vi "Host Main.vi"() -> ()   [LabVIEW 2017]
doc: "This application launches and executes the Tag Bus Data framework configuration for the specified target alias. This is a simple example of the framework API functions, but may also be a suitable starting point for a Host UI or Thick Client that is running a local version of the framework."
uses:
  <vilib>/NI/Module Execution Interface/Engine Runtime/Execution States.ctl
  <vilib>/NI/Module Execution Interface/Engine Runtime/Fault.ctl
  <vilib>/NI/Tag Bus Module Framework/runtime/error classification.ctl
  <vilib>/NI/Current Value Table/DataTypes/Double_Read.vi
  <vilib>/NI/Current Value Table/Type to Enum.vi
  <vilib>/NI/Current Value Table/DataTypes/Double_Type To Enum.vi
  <vilib>/NI/Current Value Table/FGVs/CVT Globals.vi
  <vilib>/NI/Current Value Table/FGVs/Tag Memory.vi
  <vilib>/NI/Current Value Table/Memory Block.vi
  <vilib>/NI/Current Value Table/DataTypes/Double_Memory Block.vi
  <vilib>/NI/Module Execution Interface/Engine Runtime/Engine Runtime Interface.lvclass
  <vilib>/NI/DCAF/Tag Editor Core/Framework Configuration Classes/target runtime/PL_Target Runtime.lvclass
  <vilib>/NI/Tag Bus Module Framework/runtime/TBM module execution interface.lvclass
  <vilib>/NI/Current Value Table/Current Value Table.lvlib
panel:
  out "Value":dbl
  out "engine status":T4(array[cluster])
  in  "stop":bool
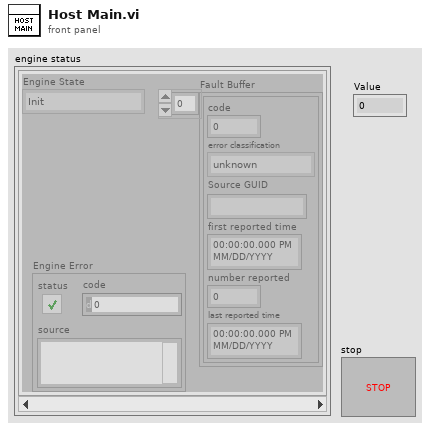
[diagram p1: front panel]
types:
  T1 = typedef "Engine Runtime Interface.lvclass/Execution States.ctl" = enum16{"Init", "Pre-Operational", "Safe-Operational", "Operational", "Stopped"}
  T2 = typedef "Engine Runtime Interface.lvclass/Fault.ctl" = cluster{"code":i32, "error classification":T3, "Source GUID":string, "first reported time":timestamp, "number reported":u32, "last reported time":timestamp}
  T3 = typedef "TBM module execution interface.lvclass/error classification.ctl" = enum16{"unknown", "none", "trivial", "recoverable", "critical"}
  T4 = cluster{"Engine State":T1, "Fault Buffer":T2[], "Engine Error":errorcluster}[]
  T5 = cluster{"Engine State":T1, "Fault Buffer":T2[], "Engine Error":errorcluster}
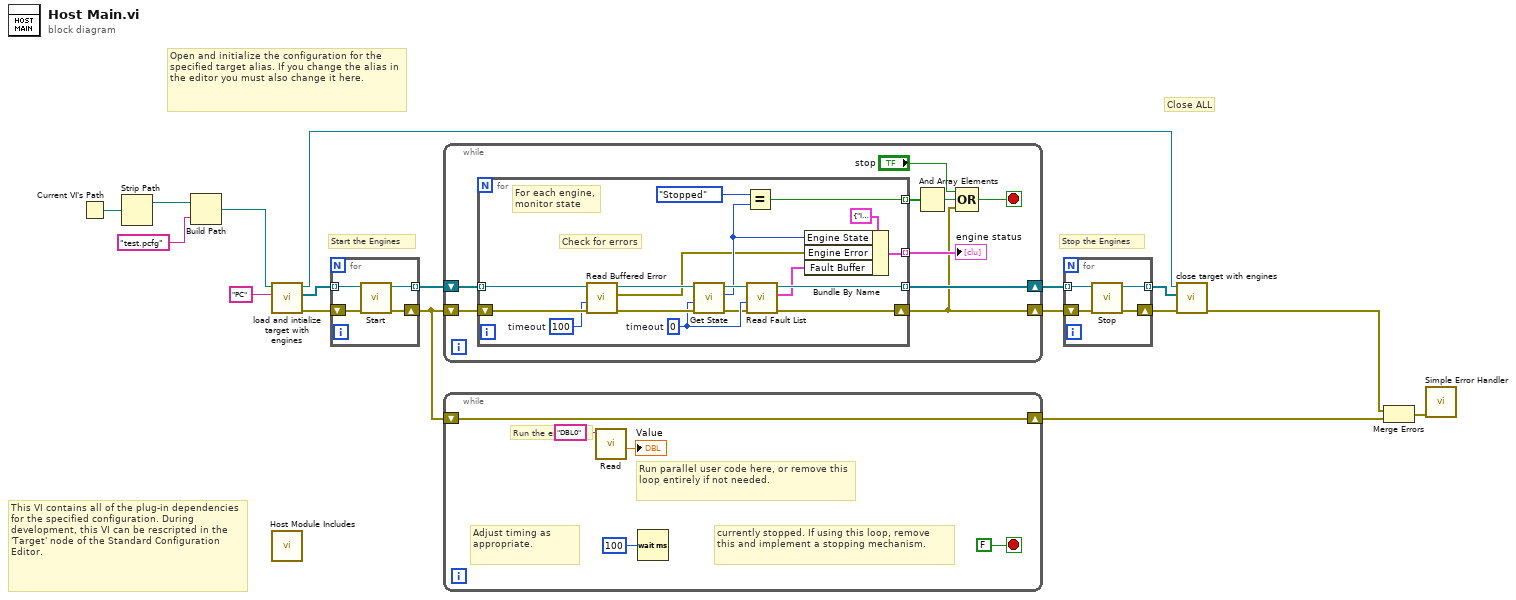
[diagram p0: block diagram]
diagram:
  # "Start the Engines"
  # "Open and initialize the configuration for the specified target alias. If you change the alias in the editor you must also change it here."
  # "Close ALL"
  # "Stop the Engines"
  # "This VI contains all of the plug-in dependencies for the specified configuration. During development, this VI can be rescripted in the 'Target' node of the Standard Configuration Editor."
  # "Run the engines"
  n1 = Current VI's Path() -> (path=w4:path)
  n2 = Strip Path(path=w4) -> (stripped path=w3:path)  [unwired: 1 out]
  n3 = Build Path(base path=w3, name or relative path="test.pcfg") -> (appended path=w2:path)
  n4 = call <vilib>:"load and intialize target with engines.vi"("target alias"="PC", "file path"=w2) -> ("error out"=w14:errorcluster, "engine runtime interfaces"=w13:refnum<class "Engine Runtime Interface.lvclass">[], "target runtime"=w10:refnum<class "PL_Target Runtime.lvclass">)  [unwired: 7 in]
  n5 = call "Host Module Includes.vi"() -> ()  [unwired: 12 in]
  n6 = for {
    tunnel: [w21] -> w17 mode=indexing
    tunnel: w13 -> [w18] mode=indexing
    shift-right: [w20] -> w8
    shift-left: w14 -> [w19]
    n7 = call-dynamic "Start.vi"("error in"=w19, "Engine Runtime Interface in"=w18) -> ("error out"=w20:errorcluster, "Engine Runtime Interface out"=w21:refnum<class "Engine Runtime Interface.lvclass">)  [unwired: 8 in]
  }
  n8 = while {
    shift-right: [w28] -> w16
    shift-left: w17 -> [w30]
    shift-right: [w22] -> w15
    shift-left: w8 -> [w29]
    stop <- w26 stop-if-true
    n9 = for {
      tunnel: w30 -> [w47] mode=indexing
      tunnel: [w39] -> w28 mode=indexing
      tunnel: [w42] -> w24 mode=indexing
      shift-right: [w38] -> w22
      shift-left: w29 -> [w46]
      tunnel: [w34] -> w25 mode=indexing
      w37 = 0  # timeout
      w41 = 100  # timeout
      # "For each engine, \nmonitor state"
      # "Check for errors"
      n10 = call-dynamic "Read Buffered Error.vi"("error in"=w46, "timeout in ms (0)"=w41, "Engine Runtime Interface in"=w47) -> ("error out"=w44:errorcluster, "Engine Error"=w32:errorcluster, "Engine Runtime Interface out"=w45:refnum<class "Engine Runtime Interface.lvclass">)  [unwired: 6 in]
      n11 = call-dynamic "Get State.vi"("error in"=w44, "timeout (-1)"=w37, "Engine Runtime Interface in"=w45) -> ("error out"=w31:errorcluster, "Engine State"=w36:T1, "Engine Runtime Interface out"=w40:refnum<class "Engine Runtime Interface.lvclass">)  [unwired: 6 in]
      n12 = Equal?(x=Execution_States."Stopped" ("Engine State"), y=w36) -> (x = y?=w42:bool)
      n13 = call-dynamic "Read Fault List.vi"("error in"=w31, "timeout (-1)"=w37, "Engine Runtime Interface in"=w40) -> ("error out"=w38:errorcluster, "faults"=w35:T2[], "Engine Runtime Interface out"=w39:refnum<class "Engine Runtime Interface.lvclass">)  [unwired: 6 in]
      n14 = Bundle By Name(cluster=T5 {"Engine State"=enum."Init", "Fault Buffer"=[], "Engine Error"={"status"=FALSE, "code"=0, "source"=""}}, "Engine State"=w36, "Engine Error"=w32, "Fault Buffer"=w35) -> (w34:T5)
    }
    "engine status" <- w25
    n15 = And Array Elements(Boolean array=w24) -> (logical AND=w23:bool)
    n16 = Compound Arithmetic op=OR("stop", w23, w22) -> (w26:bool)
  }
  n17 = while {
    shift-right: [w50] -> w7
    shift-left: w8 -> [w50]
    stop <- FALSE stop-if-true
    # "currently stopped. If using this loop, remove \nthis and implement a stopping mechanism."
    # "Adjust timing as appropriate."
    # "Run parallel user code here, or remove this loop entirely if not needed."
    n18 = call-poly <vilib>:"Read.vi"("Tag Name"="DBL0") -> ("Value"=→"Value":dbl)  [unwired: 9 in, 1 out]
    n19 = Wait (ms)(milliseconds to wait=u32 100) -> ()  [unwired: 1 out]
  }
  n20 = for {
    tunnel: w16 -> [w56] mode=indexing
    shift-right: [w53] -> w9
    shift-left: w15 -> [w55]
    tunnel: [w54] -> w11 mode=indexing
    n21 = call-dynamic "Stop.vi"("error in"=w55, "Engine Runtime Interface in"=w56) -> ("error out"=w53:errorcluster, "Engine Runtime Interface out"=w54:refnum<class "Engine Runtime Interface.lvclass">)  [unwired: 8 in]
  }
  n22 = call <vilib>:"close target with engines.vi"("error in"=w9, "Engine Runtime Interfaces"=w11, "Target Runtime"=w10) -> ("error out"=w5:errorcluster)  [unwired: 8 in]
  n23 = Merge Errors(w5, w7) -> (w6:errorcluster)
  n24 = call <vilib>:"Simple Error Handler.vi"("error in (no error)"=w6) -> ()  [unwired: 4 in, 5 out]
